vi "Generate Acquire RTDmap.vi"() -> ()   [LabVIEW 2017]
uses:
  vi.lib/UeiDaq/UeiDaqReadOneScaledScan.vi
  <vilib>/ptbypt/NI_PtbyPt.lvlib
  <resource>/objmgr/ueidaq.rc
  vi.lib/UeiDaq/UeiDaqCreateAOSession.vi
  vi.lib/UeiDaq/UeiDaqCreateAISession.vi
  vi.lib/UeiDaq/UeiDaqConfigureTimingForRTDMapIO.vi
  vi.lib/UeiDaq/UeiDaqWriteOneScaledScan.vi
panel:
  out "Number of AO channels":u32=4
  out "Number of AI channels":u32=1
  in  "AO Resource":string="pdna://192.168.100.2/Dev0/Ao0:3"
  in  "Graph Display On":bool
  in  "Sample rate":dbl=50.0
  in  "timeout (ms)":u32=2000
  in  "Analog Input Mode":enum16{"Differential", "Single-Ended"}(ring)
  in  "max. range (V)":dbl=10.0
  in  "min. range (V)":dbl=-10.0
  in  "AI Resource":string="pdna://192.168.100.2/Dev6/Ai0:3"
  out "Total scans acquired":i32
  out "Waveform Chart":dbl[][](graph)
  in  "stop":bool
  # "RTDMap analog input/output"
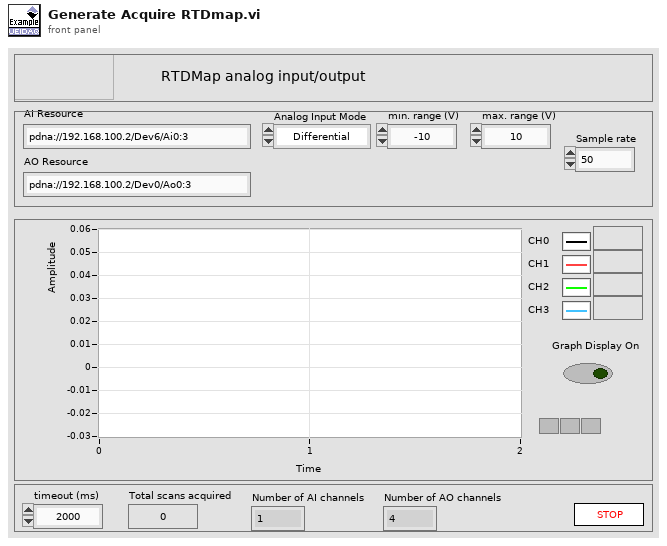
[diagram p1: front panel]
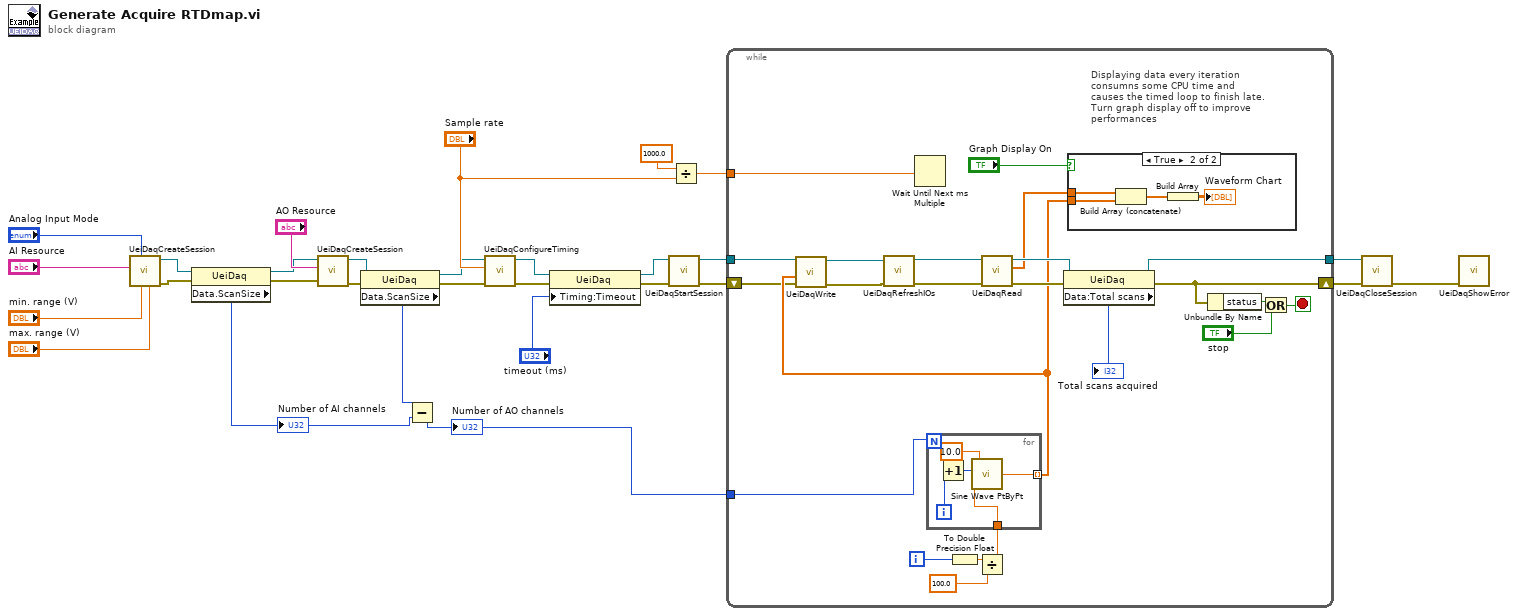
[diagram p0: block diagram]
diagram:
  n1 = call-poly "UeiDaqCreateSession.vi"("Maximum range"="max. range (V)", "Minimum range"="min. range (V)", "Analog Input Mode"="Analog Input Mode", "Resource"="AI Resource") -> ("error out"=w10:errorcluster, "UeiDaq Refnum Out"=w11:refnum<k20>)  [unwired: 2 in, 4 out]
  n2 = property class="UeiDaq"(reference=w11, error in=w10) -> (reference out=w9:refnum<k20>, error out=w8:errorcluster, "Data.ScanSize"=w3:u32)
  "Number of AI channels" <- w3
  n3 = call-poly "UeiDaqCreateSession.vi"("error in (no error)"=w8, "Resource"="AO Resource", "UeiDaq Refnum In"=w9) -> ("error out"=w4:errorcluster, "UeiDaq Refnum Out"=w5:refnum<k20>)  [unwired: 2 in, 5 out]
  n4 = property class="UeiDaq"(reference=w5, error in=w4) -> (reference out=w7:refnum<k20>, error out=w6:errorcluster, "Data.ScanSize"=w2:u32)
  n5 = Subtract(x=w2, y=w3) -> (x-y=w1:u32)
  "Number of AO channels" <- w1
  n6 = call-poly "UeiDaqConfigureTiming.vi"("error in (no error)"=w6, "Rate"="Sample rate", "UeiDaq Refnum In"=w7) -> ("error out"=w25:errorcluster, "UeiDaq Refnum Out"=w24:refnum<k20>)  [unwired: 7 out]
  n7 = property class="UeiDaq"(reference=w24, error in=w25, "Timing:Timeout"="timeout (ms)") -> (reference out=w14:refnum<k20>, error out=w15:errorcluster)
  n8 = call "UeiDaqStartSession.vi"("error in (no error)"=w15, "UeiDaq Refnum In"=w14) -> ("error out"=w12:errorcluster, "UeiDaq Refnum Out"=w13:refnum<k20>)  [unwired: 8 out]
  n9 = Divide(x=1000.0, y="Sample rate") -> (x/y=w19:dbl)
  n10 = while {
    tunnel: w13 -> [w35]
    tunnel: [w47] -> w20
    shift-right: [w36] -> w21
    shift-left: w12 -> [w34]
    tunnel: w1 -> [w40]
    tunnel: w19 -> [w37]
    i -> [w41]
    stop <- w50 stop-if-true
    # "Displaying data every iteration\nconsumns some CPU time and\ncauses the timed loop to finish late.\nTurn graph display off to improve\nperformances"
    n11 = Wait Until Next ms Multiple(millisecond multiple=w37) -> ()  [unwired: 1 out]
    n12 = To Double Precision Float(number=w41) -> (double precision float=w42:dbl)
    n13 = Divide(x=w42, y=100.0) -> (x/y=w39:dbl)
    n14 = for {
      N: w40 -> [_]
      tunnel: w39 -> [w57]
      tunnel: [w53] -> w38 mode=indexing
      i -> [w55]
      n15 = Increment(x=w55) -> (x+1=w56:i32)
      n16 = call <vilib>:"Sine Wave PtByPt.vi"("time"=w57, "frequency"=w56, "amplitude"=10.0) -> ("sine wave"=w53:dbl)  [unwired: 1 in]
    }
    n17 = call-poly "UeiDaqWrite.vi"("error in (no error)"=w34, "Scaled Data"=w38, "UeiDaq Refnum In"=w35) -> ("error out"=w32:errorcluster, "UeiDaq Refnum Out"=w33:refnum<k20>)  [unwired: 7 out]
    n18 = call "UeiDaqRefreshIOs.vi"("error in (no error)"=w32, "UeiDaq Refnum In"=w33) -> ("error out"=w30:errorcluster, "UeiDaq Refnum Out"=w31:refnum<k20>)  [unwired: 8 in]
    n19 = call-poly "UeiDaqRead.vi"("error in (no error)"=w30, "UeiDaq Refnum In"=w31) -> ("error out"=w48:errorcluster, "Scaled Data"=w45:dbl[], "UeiDaq Refnum Out"=w49:refnum<k20>)  [unwired: 7 out]
    n20 = property class="UeiDaq"(reference=w49, error in=w48) -> (reference out=w47:refnum<k20>, error out=w36:errorcluster, "Data:Total scans"=→"Total scans acquired":u32)
    n21 = case shown="True" "Graph Display On" {
      tunnel: w45 -> [_ w60]
      tunnel: w38 -> [_ w58]
      frame False {
      }
      frame True {
        n22 = Build Array (concatenate)(w60, w58) -> (w59:dbl[])
        n23 = Build Array(w59) -> (→"Waveform Chart":dbl[][])
      }
    }
    n24 = Unbundle By Name(w36) -> ("status"=w52:bool)
    n25 = Or(x=w52, y="stop") -> (x .or. y?=w50:bool)
  }
  n26 = call "UeiDaqCloseSession.vi"("error in (no error)"=w21, "UeiDaq Refnum In"=w20) -> ("error out"=w18:errorcluster)  [unwired: 1 in, 8 out]
  n27 = call "UeiDaqShowError.vi"("error in (no error)"=w18) -> ()  [unwired: 2 in, 9 out]
